vi "python.vi"() -> ()   [LabVIEW 2020]
panel:
  in  "error in (no error)":errorcluster
  out "Return value":u32
  out "error out":errorcluster
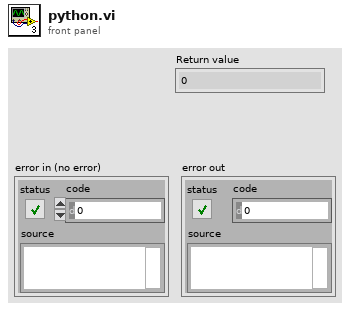
[diagram p1: front panel]
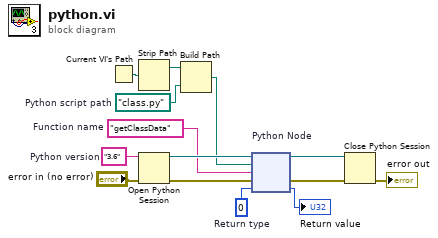
[diagram p0: block diagram]
diagram:
  w2 = path "class.py"  # Python script path
  w5 = "3.6"  # Python version
  w6 = u32 0  # Return type
  w11 = "getClassData"  # Function name
  n1 = Current VI's Path() -> (path=w4:path)
  n2 = Strip Path(path=w4) -> (stripped path=w3:path)  [unwired: 1 out]
  n3 = Open Python Session(python version=w5, 3:"error in (no error)") -> (session out=w13:refnum<k35>, error out=w12:errorcluster)  [unwired: 1 in]
  n4 = Build Path(base path=w3, name or relative path=w2) -> (appended path=w1:path)
  n5 = node "Python Node"(w13, w1, w11, w12, w6) -> (w10:refnum<k35>, w9:errorcluster, →"Return value":u32)  [unwired: 2 out]
  n6 = Close Python Session(session in=w10, error in=w9) -> (11:→"error out":errorcluster)
